vi "Read Measure.vi"   [LabVIEW 2022 SP3, in "Bronkhorst FLOW-BUS.lvlib"]
doc: "Reads the measured value in the selected instrument, for a direct measurement select Direct and for a percentage measurement select Percentage."
uses:
  Bronkhorst FLOW-BUS.lvlib
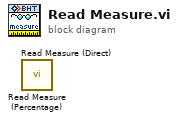
[diagram p0: block diagram]
diagram:
  n1 = call "Read Measure (Percentage).vi"() -> ()  [unwired: 9 in, 3 out]
  n2 = call "Read Measure (Direct).vi"() -> ()  [unwired: 9 in, 3 out]
